vi "projekt_pomoc2.vi"(9 "String 2":string, 10 "String":string, 11 "Boolean":bool) -> (2 "String 3":string)   [LabVIEW 2023]
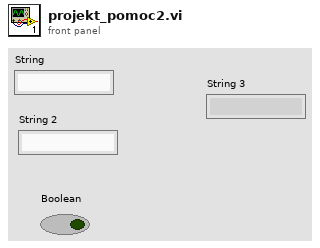
[diagram p1: front panel]
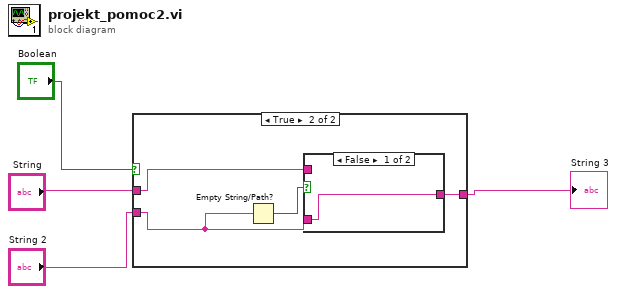
[diagram p0: block diagram]
diagram:
  n1 = case shown="True" "Boolean" {
    tunnel: "String" -> [_ w8]
    tunnel: "String 2" -> [w5 w7]
    tunnel: [w5 w6] -> w1
    frame False {
    }
    frame True {
      n2 = Empty String/Path?(string/path=w7) -> (empty?=w9:bool)
      n3 = case shown="False" w9 {
        tunnel: w8 -> [_ w11]
        tunnel: w7 -> [w10 _]
        tunnel: [w10 w11] -> w6
        frame False {
        }
        frame True {
        }
      }
    }
  }
  "String 3" <- w1
